vi "Read Attributes.vi"(11 "Result Msg":refnum<class "Result Msg.lvclass">) -> (2 "Payload":cluster{"Json Result":string})   [LabVIEW 2021, in "Inference.lvlib" / "Result Msg.lvclass"]
uses:
  Result Msg.lvclass
  Result Msg.lvclass/Result Msg.ctl
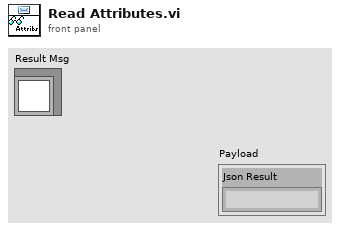
[diagram p1: front panel]
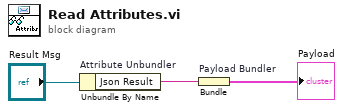
[diagram p0: block diagram]
diagram:
  n1 = Unbundle By Name "Attribute Unbundler"("Result Msg") -> ("Json Result"=w1:string)
  n2 = Bundle "Payload Bundler"("Json Result"=w1) -> (→"Payload":cluster{"Json Result":string})  [unwired: 1 in]
